vi "[RT]Read_I2C.vi"(8 "error in (no error)":errorcluster) -> (1 "Druck (bar)":dbl format="%.7f", 2 "Luftfeuchtigkeit %rH":dbl format="%.7f", 3 "Temp (°C)":dbl format="%.7f")   [LabVIEW 2018]
doc: "The myRIO Project template acquires acceleration data from the onboard accelerometer and displays the changes of acceleration values in a waveform chart."
uses:
  <vilib>/myRIO/Instrument Drivers/Onboard IO/I2C/typedefs/I2C User Configuration.ctl
  <vilib>/myRIO/Instrument Drivers/Onboard IO/I2C/typedefs/I2C Transfer Rate.ctl
  <vilib>/myRIO/Instrument Drivers/Onboard IO/DIO/typedefs/DIO Reference.ctl
  <vilib>/myRIO/Common/Instrument Driver Framework/Utilities/typedefs/myRIO Generic Hardware Reference.ctl
  <vilib>/myRIO/Common/Instrument Driver Framework/Utilities/typedefs/Hardware Version Enum.ctl
  <vilib>/myRIO/Common/Instrument Driver Framework/Utilities/typedefs/myRIO v1.0 Reference.ctl
  <vilib>/myRIO/Common/Instrument Driver Framework/Utilities/typedefs/Generic FPGA Reference.ctl
  <vilib>/myRIO/Common/Instrument Driver Framework/myRIO v1.0/DIO/typedefs/DIO Channels List.ctl
  <vilib>/myRIO/Common/Instrument Driver Framework/myRIO v1.0/DIO/typedefs/DIO Channels Enum.ctl
  <vilib>/userdefined/High Color/nirio_resource_hc.ctl
  <vilib>/myRIO/Instrument Drivers/Onboard IO/I2C/typedefs/I2C Reference.ctl
  <vilib>/myRIO/Common/Instrument Driver Framework/myRIO v1.0/I2C/typedefs/I2C Channels Enum.ctl
  <vilib>/myRIO/Instrument Drivers/Onboard IO/I2C/typedefs/I2C Configuration.ctl
  <vilib>/myRIO/Common/Instrument Driver Framework/myRIO v1.0/DIO/vis/myRIO v1.1 Open DIO.vi
  <vilib>/myRIO/Common/Instrument Driver Framework/myRIO v1.0/I2C/vis/myRIO v1.1 Open I2C.vi
  <vilib>/myRIO/Common/Instrument Driver Framework/Utilities/vis/Validate Channels.vi
  <vilib>/myRIO/Common/Instrument Driver Framework/myRIO v1.0/DIO/vis/myRIO v1.0 Reserve DIO.vi
  <vilib>/myRIO/Common/Instrument Driver Framework/myRIO v1.0/I2C/vis/myRIO v1.0 Reserve I2C.vi
  <vilib>/myRIO/Common/Instrument Driver Framework/myRIO v1.0/I2C/vis/myRIO v1.0 Close I2C.vi
  <vilib>/myRIO/Common/Instrument Driver Framework/myRIO v1.0/DIO/vis/myRIO v1.0 Close DIO.vi
  <vilib>/myRIO/Common/Instrument Driver Framework/myRIO v1.0/Resource Manager/vis/myRIO v1.0 Reserve Channel List.vi
  <vilib>/myRIO/Common/Instrument Driver Framework/myRIO v1.0/DIO/vis/myRIO v1.0 Build MUX Configuration DIO.vi
  <vilib>/myRIO/Common/Instrument Driver Framework/myRIO v1.0/I2C/vis/myRIO v1.0 Build MUX Configuration I2C.vi
  <vilib>/myRIO/Common/Instrument Driver Framework/myRIO v1.0/I2C/vis/myRIO v1.0 Unreserve I2C.vi
  <vilib>/myRIO/Common/Instrument Driver Framework/myRIO v1.0/DIO/vis/myRIO v1.0 Unreserve DIO.vi
  <vilib>/myRIO/Common/Instrument Driver Framework/myRIO v1.0/Resource Manager/vis/myRIO v1.0 Reserve Channel.vi
  <vilib>/myRIO/Common/Instrument Driver Framework/myRIO v1.0/Resource Manager/vis/myRIO v1.0 Unreserve Channel.vi
  <vilib>/myRIO/Common/Instrument Driver Framework/myRIO v1.0/Resource Manager/vis/myRIO v1.0 Create Configuration List.vi
  <vilib>/myRIO/Common/Instrument Driver Framework/myRIO v1.0/Resource Manager/vis/myRIO v1.0 Unreserve Channel List.vi
  <vilib>/myRIO/Common/Instrument Driver Framework/myRIO v1.0/Resource Manager/vis/myRIO v1.0 Build Mutex Name.vi
  <vilib>/Utility/VariantDataType/GetNumericInfo.vi
  <vilib>/Utility/error.llb/Error Cluster From Error Code.vi
  <vilib>/myRIO/Common/Instrument Driver Framework/myRIO v1.0/myRIO v1.1 Open.vi
  <vilib>/myRIO/Common/Instrument Driver Framework/Utilities/vis/IO Manager.vi
  <vilib>/myRIO/Common/Instrument Driver Framework/Utilities/vis/Configuration Manager.vi
  <vilib>/myRIO/Common/Instrument Driver Framework/myRIO v1.0/Resource Manager/vis/myRIO v1.0 Configure IO.vi
  <vilib>/myRIO/Common/Instrument Driver Framework/myRIO v1.0/myRIO v1.0 Close.vi
  <vilib>/myRIO/Common/Instrument Driver Framework/myRIO v1.0/I2C/vis/myRIO v1.0 Configure I2C.vi
  [GlobVar]SensorState.vi
  <vilib>/myRIO/Common/Instrument Driver Framework/myRIO v1.0/I2C/vis/myRIO v1.0 Read I2C.vi
  <vilib>/myRIO/Common/Instrument Driver Framework/myRIO v1.0/I2C/vis/myRIO v1.0 Shutdown I2C.vi
  <vilib>/myRIO/Common/Instrument Driver Framework/myRIO v1.0/DIO/vis/myRIO v1.0 Shutdown DIO.vi
  <vilib>/myRIO/Instrument Drivers/Onboard IO/I2C/vis/myRIO I2C Open.xnode
  <vilib>/myRIO/Instrument Drivers/Onboard IO/DIO/vis/myRIO DIO Open.xnode
  <vilib>/myRIO/Instrument Drivers/Onboard IO/I2C/I2C.lvlib
  <vilib>/myRIO/Instrument Drivers/Onboard IO/DIO/DIO.lvlib
panel:
  out "ACK data":u8[](array[numeric]) format="%02x"
  out "UID":string
  out "# of tags":u8
  out "Bytes Read":u8[](array[numeric]) format="%02x"
  out "error out 2":errorcluster
  out "NFC erkannt":bool=TRUE
  out "State":string
  out "Bytes Read Config":u8[](array[numeric]) format="%02x"
  out "ACK Config":bool
  out "Timeout occured?":bool
  out "ADC RAW PRESSURE":u32 format="%020b"
  out "Bytes Read Pressure":u8[](array[numeric]) format="%08b"
  out "Bytes Read Humidity":u8[](array[numeric]) format="%08b"
  out "ADC RAW HUMIDITY":u32 format="%016b"
  out "ADC RAW TEMP":i32 format="%020b"
  out "Bytes Read Temp":u8[](array[numeric]) format="%08b"
  out "ChipID":u8[](array[numeric]) format="%x"
  # "BME280"
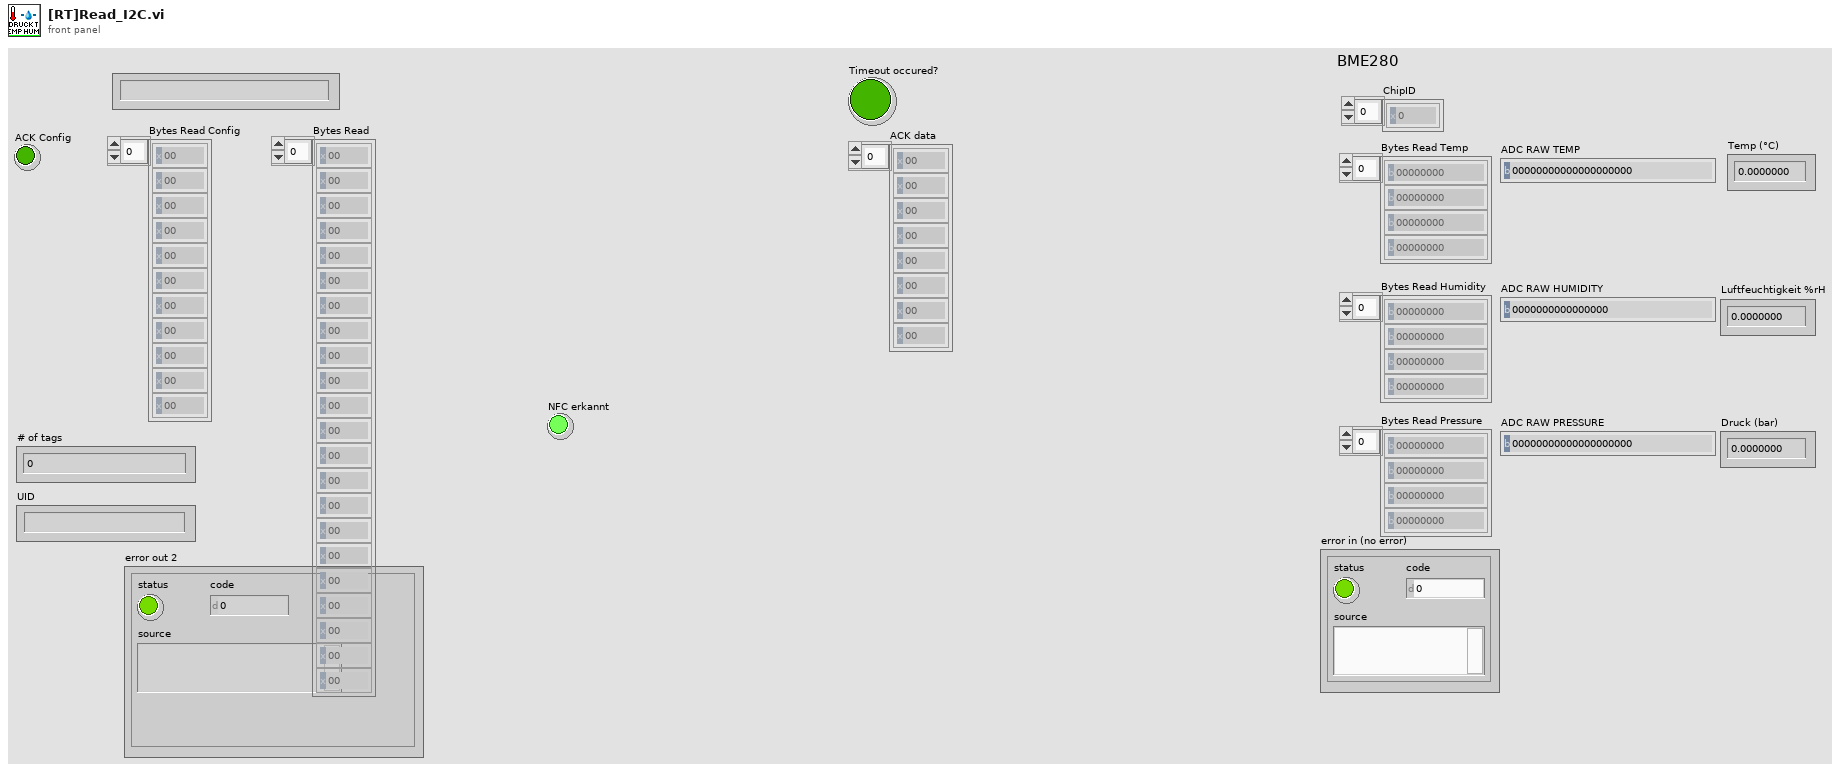
[diagram p1: front panel]
types:
  T1 = typedef "I2C.lvlib/I2C User Configuration.ctl" = cluster{"I2C Transfer Rate":T2}
  T2 = typedef "I2C.lvlib/I2C Transfer Rate.ctl" = enum16{"Standard mode (100 kbps)", "Fast mode (400 kbps)"}
  T3 = typedef "I2C.lvlib/I2C Reference.ctl" = cluster{"myRIO Reference":T4, "I2C Channels Enum":T8, "I2C Configuration":T9}
  T4 = typedef "myRIO Generic Hardware Reference.ctl" = cluster{"myRIO Model":T5, "myRIO Hardware Reference":T6}
  T5 = typedef "Hardware Version Enum.ctl" = enum16{"Unknown", "myRIO-1900", "myRIO-1950", "roboRIO", "NI ELVIS RIO CM", "ELVIS III"}
  T6 = typedef "myRIO v1.0 Reference.ctl" = cluster{"Generic FPGA Reference":T7, "Allow multiple opens":bool}
  T7 = typedef "Generic FPGA Reference.ctl" = refnum<k20>
  T8 = typedef "I2C Channels Enum.ctl" = enum16{"Not Connected", "A/I2C", "B/I2C", "I2C/I2C"}
  T9 = typedef "I2C.lvlib/I2C Configuration.ctl" = cluster{"I2C Transfer Rate":T2}
  T10 = typedef "DIO.lvlib/DIO Reference.ctl" = cluster{"myRIO Reference":T4, "DIO Channels List":T11}
  T11 = typedef "DIO Channels List.ctl" = T12[]
  T12 = typedef "DIO Channels Enum.ctl" = enum16{"Not Connected", "C/DIO0", "C/DIO1", "C/DIO2", "C/DIO3", "C/DIO4", "C/DIO5", "C/DIO6", "C/DIO7", "A/DIO0", "A/DIO1", "A/DIO2", "A/DIO3", "A/DIO4", "A/DIO5", "A/DIO6", "A/DIO7", "A/DIO8", "A/DIO9", "A/DIO10", "A/DIO11", "A/DIO12", "A/DIO13", "A/DIO14", "A/DIO15", "A/DIO16", "A/DIO17", "A/DIO18", "A/DIO19", "B/DIO0", "B/DIO1", "B/DIO2", "B/DIO3", "B/DIO4", "B/DIO5", "B/DIO6", "B/DIO7", "B/DIO8", "B/DIO9", "B/DIO10", "B/DIO11", "B/DIO12", "B/DIO13", "B/DIO14", "B/DIO15", "B/DIO16", "B/DIO17", "B/DIO18", "B/DIO19", "LED0", "LED1", "LED2", "LED3", "Button0", "DIO/DIO0", "DIO/DIO1", "DIO/DIO2", "DIO/DIO3", "DIO/DIO4", "DIO/DIO5", "DIO/DIO6", "DIO/DIO7", "DIO/DIO8", "DIO/DIO9", "SPI/CS0", "SPI/CS1", "SPI/CS2", "SPI/CS3", "LED RADIO (Green)", "LED RADIO (Red)", "LED COMM (Green)", "LED COMM (Red)", "LED MODE (Green)", "LED MODE (Red)"}
  T13 = typedef "calib_data.ctl" = cluster{"dig_T1":u16, "dig_T2":i16, "dig_T3":i16, "dig_P1":u16, "dig_P2":i16, "dig_P3":i16, "dig_P4":i16, "dig_P5":i16, "dig_P6":i16, "dig_P7":i16, "dig_P8":i16, "dig_P9":i16, "dig_H1":u8, "dig_H2":i16, "dig_H3":u8, "dig_H4":i16, "dig_H5":i16, "dig_H6":i8}
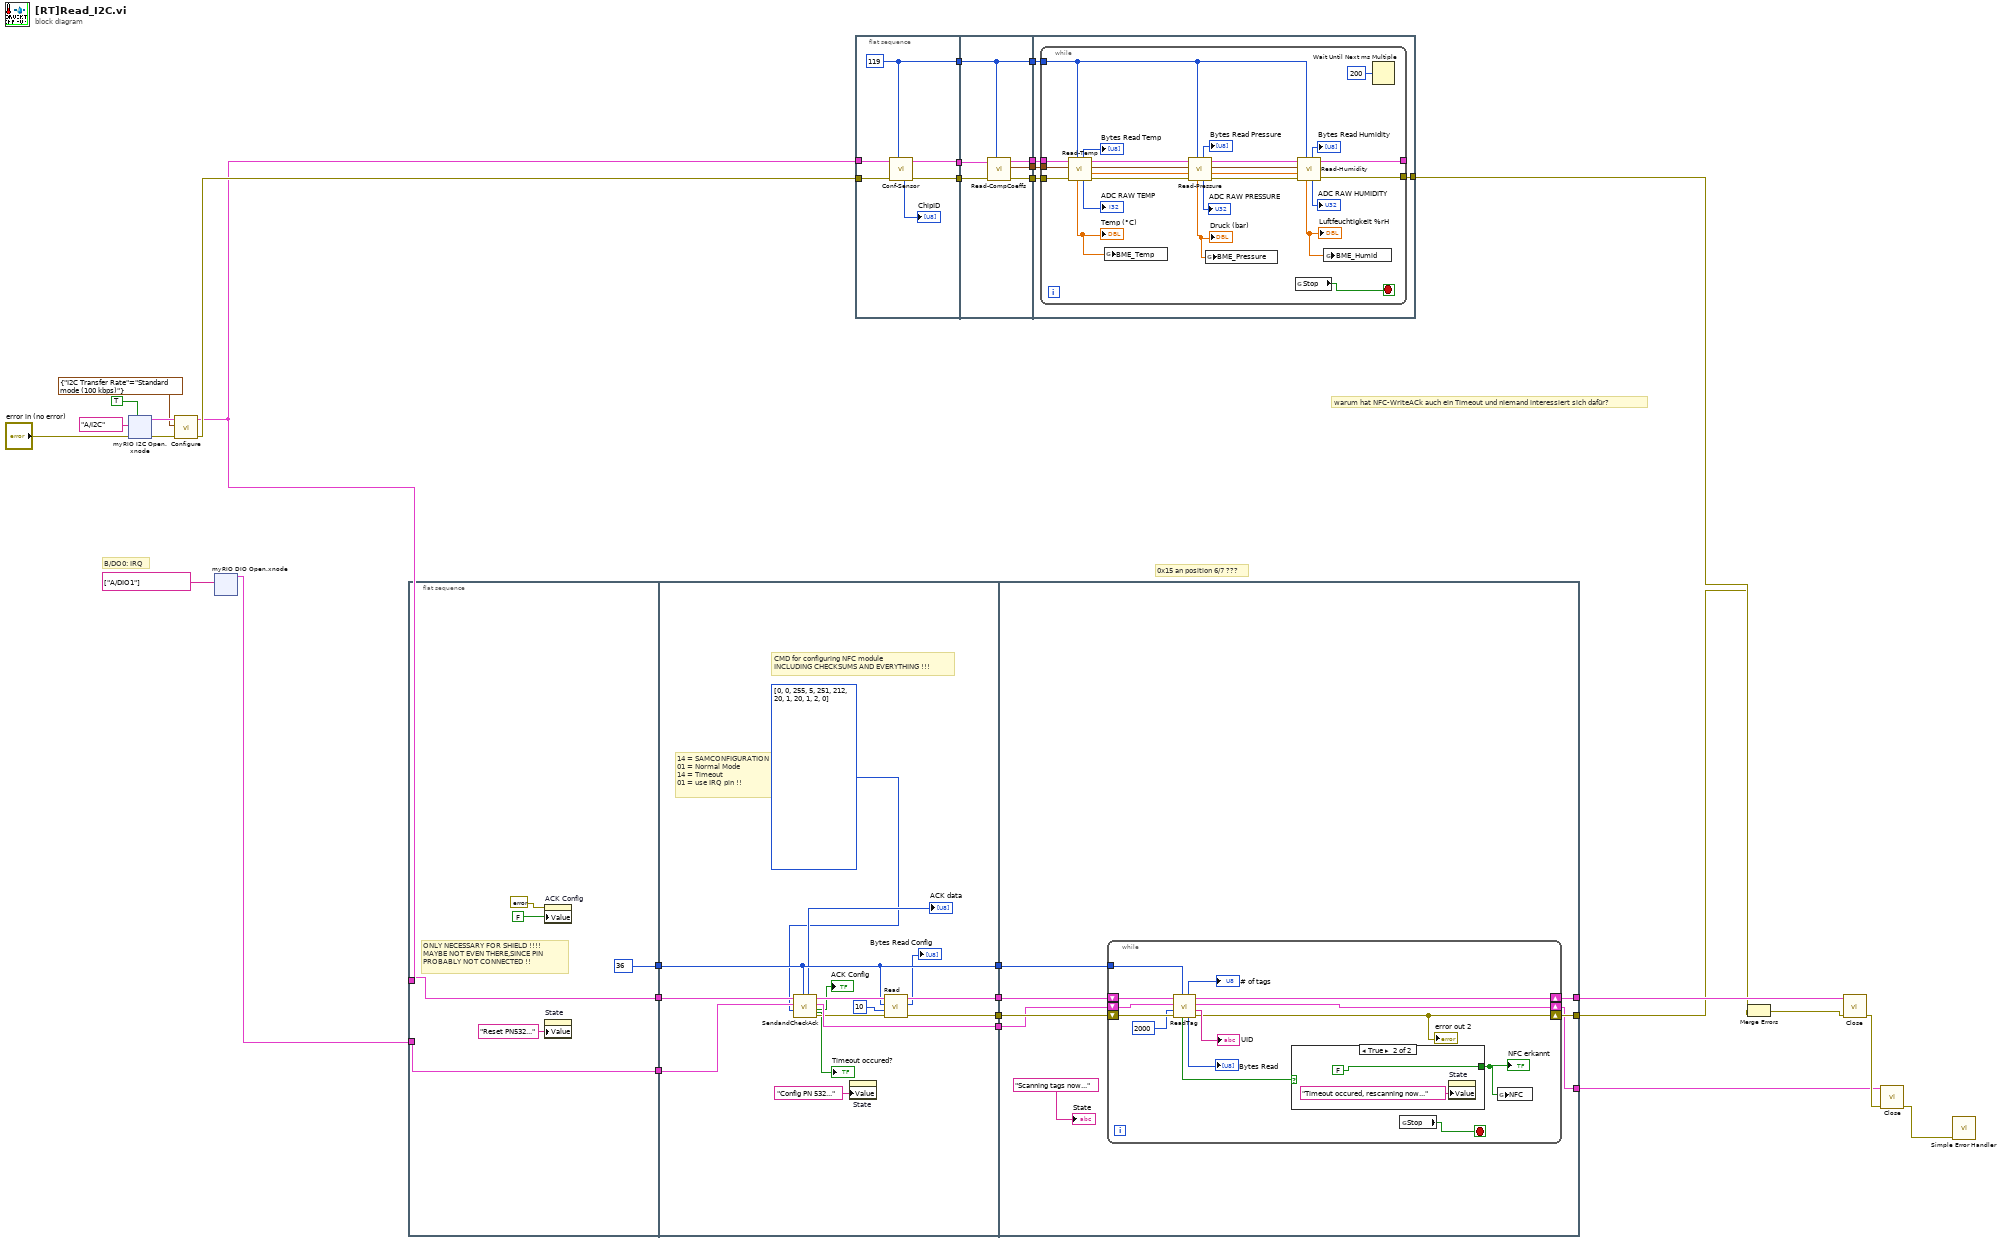
[diagram p0: block diagram]
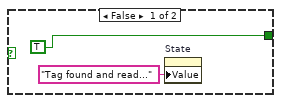
[diagram p2: hidden frame]
diagram:
  # "B/DO0: IRQ"
  # "warum hat NFC-WriteACk auch ein Timeout und niemand interessiert sich dafür?"
  # "0x15 an position 6/7 ???"
  n1 = xnode "myRIO I2C Open.xnode"("error in (no error)"="error in (no error)", "Allow multiple opens?"=TRUE, "Channel Name"=tag "A/I2C") -> ("error out"=w23:errorcluster, "I2C Ref Out"=w22:T3)
  n2 = call <vilib>:"Configure.vi"("error in (no error)"=w23, "I2C User Configuration"=T1 {"I2C Transfer Rate"=enum."Standard mode (100 kbps)"}, "I2C Ref In"=w22) -> ("error out"=w18:errorcluster, "I2C Ref Out"=w5:T3)  [unwired: 7 in]
  n3 = xnode "myRIO DIO Open.xnode"("Channel Names"=tag[] ["A/DIO1"]) -> ("DIO Ref Out"=w4:T10)  [unwired: 2 in, 1 out]
  n4 = flat-sequence {
    tunnel: [u8 36 ("Slave Address (7-bit)")] -> w17
    tunnel: [w35] -> w16
    tunnel: [w34] -> w15
    tunnel: w5 -> [w35]
    tunnel: w4 -> [w34]
    tunnel: w17 -> [w47]
    tunnel: w16 -> [w52]
    tunnel: w15 -> [w51]
    tunnel: [w50] -> w14
    tunnel: [w47] -> w13
    tunnel: [w48] -> w12
    tunnel: [w44] -> w11
    tunnel: w14 -> [w58]
    tunnel: w13 -> [w57]
    tunnel: w12 -> [w59]
    tunnel: w11 -> [w60]
    tunnel: [w56] -> w9
    tunnel: [w55] -> w2
    tunnel: [w54] -> w8
    frame #0 {
      # "ONLY NECESSARY FOR SHIELD !!!!\nMAYBE NOT EVEN THERE,SINCE PIN\nPROBABLY NOT CONNECTED !!"
      n5 = property on="ACK Config" class="Bool (strict)"(error in=errorcluster {"status"=FALSE, "code"=0, "source"=""} ("error out"), "Value"=FALSE ("ACK Config")) -> ()  [unwired: 1 in, 2 out]
      n6 = property on="State" class="Str"("Value"="Reset PN532..." ("State")) -> ()  [unwired: 2 in, 2 out]
    }
    frame #1 {
      # "CMD for configuring NFC module\nINCLUDING CHECKSUMS AND EVERYTHING !!!"
      # "14 = SAMCONFIGURATION\n01 = Normal Mode\n14 = Timeout\n01 = use IRQ pin !!"
      n7 = call "SendandCheckAck.vi"("Slave Address (7-bit)"=w47, "bytes to send"=u8[] [0, 0, 255, 5, 251, 212, 20, 1, 20, 1, 2, 0], "DI Ref In"=w51, "I2C Ref In"=w52) -> ("error out"=w46:errorcluster, "ACK?"=→"ACK Config":bool, "DI Ref Out"=w50:T10, "I2C Ref Out"=w49:T3, "Timeout occured?"=→"Timeout occured?":bool, "ACK data"=→"ACK data":u8[])  [unwired: 2 in]
      n8 = property on="State" class="Str"("Value"="Config PN 532..." ("State")) -> ()  [unwired: 2 in, 2 out]
      n9 = call <vilib>:"Read.vi"("error in (no error)"=w46, "Byte Count"=u32 10, "Slave Address (7-bit)"=w47, "I2C Ref In"=w49) -> ("error out"=w44:errorcluster, "Bytes Read"=→"Bytes Read Config":u8[], "I2C Ref Out"=w48:T3)  [unwired: 4 in]
    }
    frame #2 {
      n10 = while {
        tunnel: w57 -> [w71]
        shift-right: [w65] -> w55
        shift-left: w60 -> [w74]
        shift-right: [w66] -> w56
        shift-left: w59 -> [w73]
        shift-right: [w64] -> w54
        shift-left: w58 -> [w72]
        stop <- w62 stop-if-true
        n11 = call "ReadTag.vi"("Slave Address (7-bit)"=w71, "error in (no error)"=w74, "Timeout (ms)"=2000 ("Timeout (n-times 10 ms)"), "DI Ref Out"=w72, "I2C Ref Out in"=w73) -> ("error out"=w65:errorcluster, "UID"=→"UID":string, "DIO Ref Out out"=w64:T10, "I2C Ref Out out"=w66:T3, "Bytes Read"=→"Bytes Read":u8[], "# of tags"=→"# of tags":u8, "Timeout READ"=w63:bool)
        "error out 2" <- w65
        n12 = case shown="True" w63 {
          tunnel: [TRUE FALSE] -> w61
          frame False {
            n13 = property on="State" class="Str"("Value"="Tag found and read..." ("State")) -> ()  [unwired: 2 in, 2 out]
          }
          frame True {
            n14 = property on="State" class="Str"("Value"="Timeout occured, rescanning now..." ("State")) -> ()  [unwired: 2 in, 2 out]
          }
        }
        "NFC erkannt" <- w61
        n15 = global read "[GlobVar]SensorState.vi" "Stop"() -> (w62:bool)
        n16 = global write "[GlobVar]SensorState.vi" "NFC"(w61) -> ()
      }
      "State" <- "Scanning tags now..." ("State")
    }
  }
  n17 = flat-sequence {
    tunnel: [w84] -> w31
    tunnel: [w82] -> w30
    tunnel: [w80] -> w25
    tunnel: w5 -> [w81]
    tunnel: w18 -> [w83]
    tunnel: w31 -> [w90]
    tunnel: w30 -> [w87]
    tunnel: [w87] -> w29
    tunnel: [w89] -> w28
    tunnel: [w88] -> w27
    tunnel: [w86] -> w26
    tunnel: w25 -> [w85]
    tunnel: w29 -> [w95]
    tunnel: w28 -> [w94]
    tunnel: w27 -> [w93]
    tunnel: w26 -> [w92]
    tunnel: [w91] -> w3
    frame #0 {
      w82 = u8 119 ("Slave Address (7-bit)")
      n18 = call "Conf-Sensor.vi"("Slave Address (7-bit)"=w82, "error in (no error)"=w83, "I2C Ref Out in"=w81) -> ("error out"=w84:errorcluster, "I2C Ref Out out"=w80:T3, "ChipID"=→"ChipID":u8[])  [unwired: 6 in]
    }
    frame #1 {
      n19 = call "Read-CompCoeffs.vi"("Slave Address (7-bit)"=w87, "error in (no error)"=w90, "I2C Ref Out in"=w85) -> ("error out"=w88:errorcluster, "Comp Coeffs Out"=w86:T13, "I2C Ref Out out"=w89:T3)  [unwired: 6 in]
    }
    frame #2 {
      n20 = while {
        tunnel: w95 -> [w105]
        tunnel: w94 -> [w119]
        tunnel: w93 -> [w118]
        tunnel: w92 -> [w117]
        tunnel: [w102] -> _
        tunnel: [w101] -> w91
        stop <- w99 stop-if-true
        n21 = call "Read-Temp.vi"("Slave Address (7-bit)"=w105, "error in (no error)"=w118, "Comp Coeffs"=w117, "I2C Ref Out in"=w119) -> ("error out"=w112:errorcluster, "T_fine"=w113:dbl, "Comp Coeffs Out"=w114:T13, "I2C Ref Out out"=w115:T3, "ADC RAW TEMP"=→"ADC RAW TEMP":i32, "Bytes Read Temp"=→"Bytes Read Temp":u8[], "T"=w98:dbl)  [unwired: 1 in]
        "Temp (°C)" <- w98
        n22 = global write "[GlobVar]SensorState.vi" "BME_Temp"(w98) -> ()
        n23 = call "Read-Pressure.vi"("Slave Address (7-bit)"=w105, "error in (no error)"=w112, "T_fine"=w113, "Comp Coeffs"=w114, "I2C Ref Out in"=w115) -> ("error out"=w109:errorcluster, "T_fine Out"=w106:dbl, "Comp Coeffs Out"=w107:T13, "I2C Ref Out"=w108:T3, "ADC RAW PRESSURE"=→"ADC RAW PRESSURE":u32, "Bytes Read"=→"Bytes Read Pressure":u8[], "p"=w97:dbl)
        "Druck (bar)" <- w97
        n24 = global write "[GlobVar]SensorState.vi" "BME_Pressure"(w97) -> ()
        n25 = global read "[GlobVar]SensorState.vi" "Stop"() -> (w99:bool)
        n26 = call "Read-Humidity.vi"("Slave Address (7-bit)"=w105, "error in (no error)"=w109, "T_fine"=w106, "Comp Coeffs"=w107, "I2C Ref In"=w108) -> ("error out"=w101:errorcluster, "I2C Ref Out"=w102:T3, "ADC RAW HUMIDITY"=→"ADC RAW HUMIDITY":u32, "Bytes Read"=→"Bytes Read Humidity":u8[], "Humidity"=w96:dbl)  [unwired: 2 in]
        "Luftfeuchtigkeit %rH" <- w96
        n27 = global write "[GlobVar]SensorState.vi" "BME_Humid"(w96) -> ()
        n28 = Wait Until Next ms Multiple(millisecond multiple=u32 200) -> ()  [unwired: 1 out]
      }
    }
  }
  n29 = Merge Errors(w3, w2) -> (w1:errorcluster)
  n30 = call <vilib>:"Close.vi"("error in (no error)"=w1, "I2C Ref In"=w9) -> ("error out"=w10:errorcluster)  [unwired: 9 in]
  n31 = call <vilib>:"Close.vi"("error in (no error)"=w10, "DIO Ref In"=w8) -> ("error out"=w7:errorcluster)  [unwired: 9 in]
  n32 = call <vilib>:"Simple Error Handler.vi"("error in (no error)"=w7) -> ()  [unwired: 4 in, 5 out]
